vi "add_duration_roslv.vi"   [LabVIEW 2014]
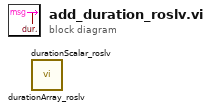
[diagram p0: block diagram]
diagram:
  n1 = call "durationArray_roslv.vi"() -> ()  [unwired: 5 in, 1 out]
  n2 = call "durationScalar_roslv.vi"() -> ()  [unwired: 5 in, 1 out]
